vi "StopProcessingLoop.vi"(8 "error in (no error)":errorcluster, 11 "navX - Interface in":refnum<class "navX - Interface.lvclass">) -> (0 "error out":errorcluster, 3 "navX - Interface out":refnum<class "navX - Interface.lvclass">)   [LabVIEW 2015, in "navX Library v3.lvlib" / "navX - Interface.lvclass"]
uses:
  navX - Interface.lvclass
  _TypeDefs/NotificationActionsTypeDef.ctl
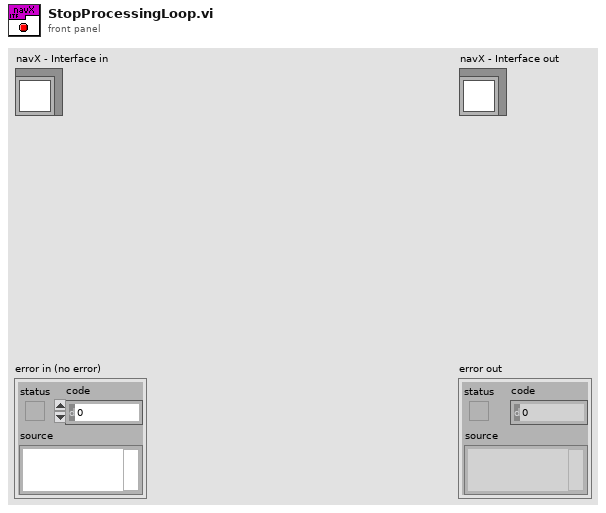
[diagram p1: front panel]
types:
  T1 = typedef "navX Library v3.lvlib/navX - Interface.lvclass/NotificationActionsTypeDef.ctl" = enum16{"UNKNOWN", "Stop Processing Loop", "Reconfigure", "Zero"}
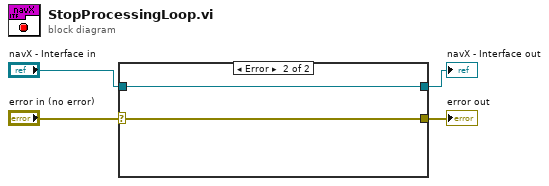
[diagram p0: block diagram]
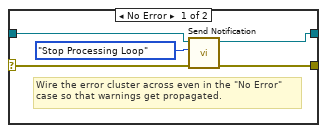
[diagram p2: hidden frame]
diagram:
  n1 = case shown="Error" "error in (no error)" {
    selector: "error in (no error)" -> [w7 w11]
    tunnel: [w6 w11] -> w3
    tunnel: [w5 w10] -> w1
    tunnel: "navX - Interface in" -> [w9 w10]
    frame No Error {
      # "Wire the error cluster across even in the \"No Error\"\ncase so that warnings get propagated."
      n2 = call "Send Notification.vi"("error in (no error)"=w7, "Notification Action"=NotificationActionsTypeDef."Stop Processing Loop", "navX - Interface in"=w9) -> ("error out"=w6:errorcluster, "navX - Interface out"=w5:refnum<class "navX - Interface.lvclass">)  [unwired: 7 in]
    }
    frame Error {
    }
  }
  "error out" <- w3
  "navX - Interface out" <- w1
